vi "PD250 - PWM test.vi"(8 "Board Selector":T1, 10 "Message IN":string=" ", 11 "HMP4040 Channel Settings":T2={"CH1 Voltage"=24.0, "CH1 Current"=1.0, "CH1 Output"=TRUE, "CH2 Voltage"=24.0, "CH2 Current"=1.0, "CH2 Output"=TRUE, "CH3 Voltage"=24.0, "CH3 Current"=1.0, "CH3 Output"=TRUE, "CH4 Voltage"=24.0, "CH4 Current"=1.0, "CH4 Output"=TRUE, "Master Output"=TRUE} {"CH4 Current" format="%.3f"; "CH4 Voltage" format="%.3f"; "CH3 Current" format="%.3f"; "CH3 Voltage" format="%.3f"; "CH2 Current" format="%.3f"; "CH2 Voltage" format="%.3f"; "CH1 Current" format="%.3f"; "CH1 Voltage" format="%.3f"}) -> (0 "error out":errorcluster, 1 "Result (bool)":bool, 2 "Message OUT":string, 3 "ControlBoard OUT":refnum<visa-resource-name>)   [LabVIEW 2022 SP3]
uses:
  HMP4000 Communication/HMP4040_ChannelControl.ctl
  Serial Board Com/Board Select.ctl
  <vilib>/DAQmx/read.llb/DAQmx Read (Analog 1D Wfm NChan NSamp).vi
  <vilib>/DAQmx/miscellaneous.llb/DAQmx Fill In Error Info.vi
panel:
  in  "error in (no error) 2":errorcluster
  out "Analysis Leg":i32
  in  "Debug Mode":bool
  out "Waveforms":T3
  out "Active Leg":i32
  out "Result (color)":u32(colorbox)
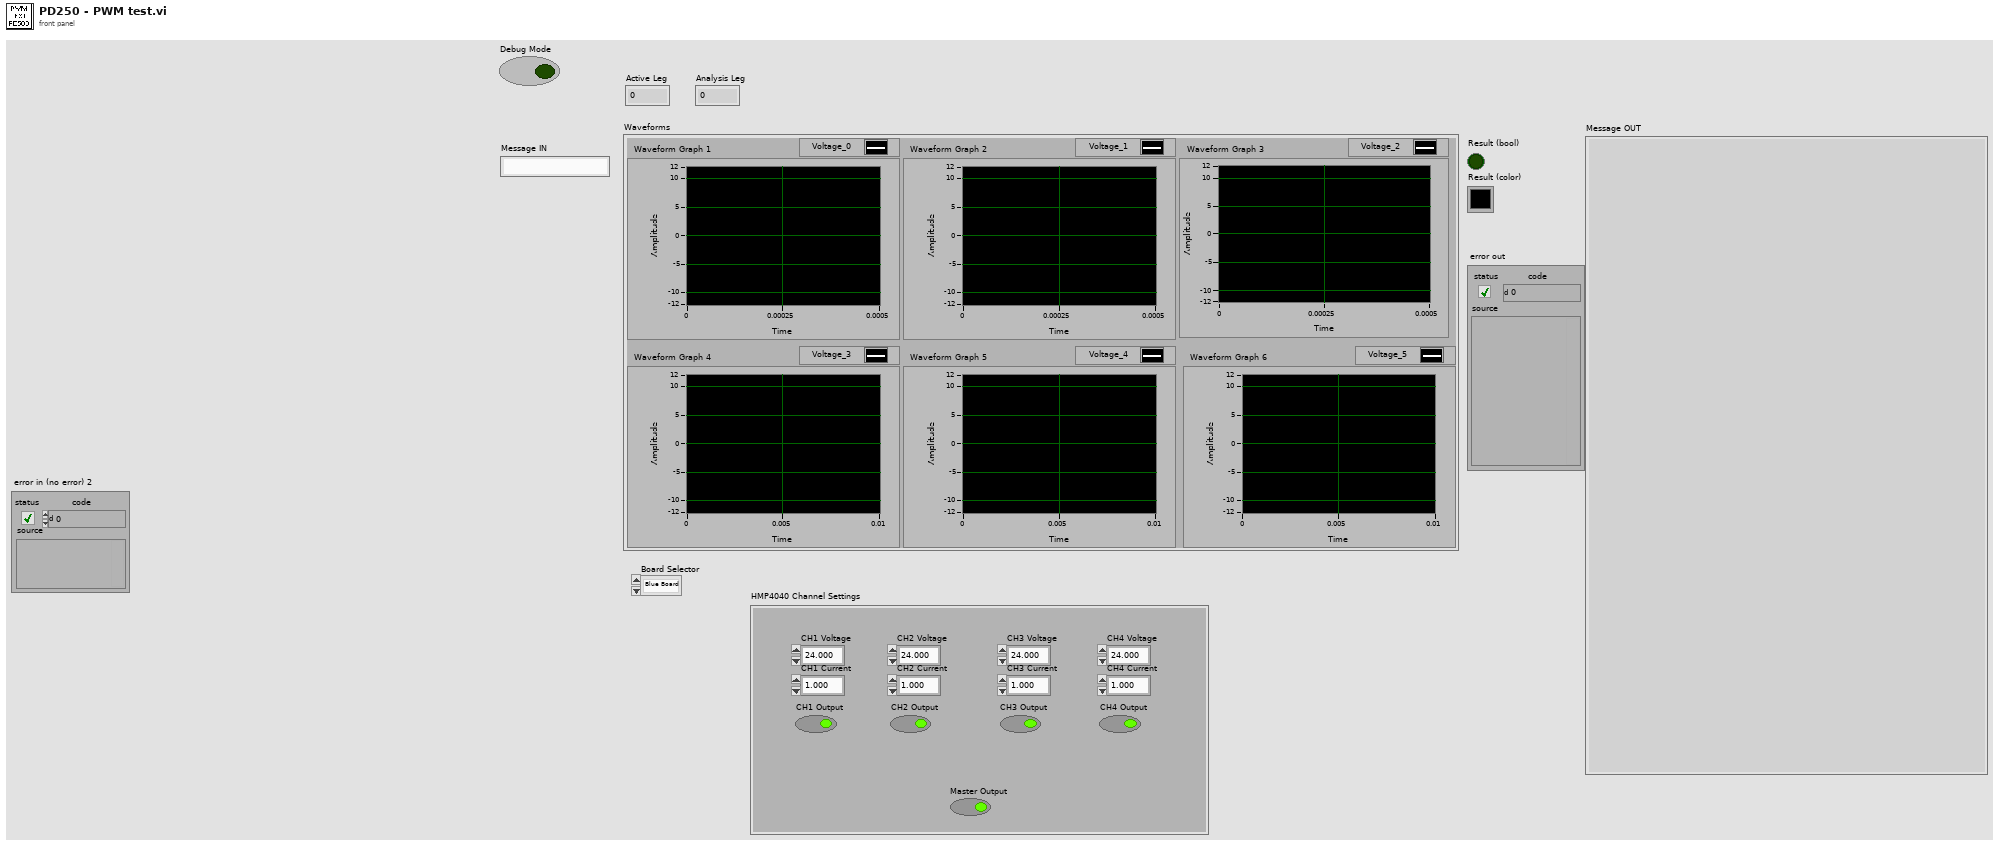
[diagram p1: front panel]
types:
  T1 = typedef "Board Select.ctl" = enum16{"Blue Board", "Green Board"}
  T2 = typedef "HMP4040_ChannelControl.ctl" = cluster{"CH1 Voltage":dbl, "CH1 Current":dbl, "CH1 Output":bool, "CH2 Voltage":dbl, "CH2 Current":dbl, "CH2 Output":bool, "CH3 Voltage":dbl, "CH3 Current":dbl, "CH3 Output":bool, "CH4 Voltage":dbl, "CH4 Current":dbl, "CH4 Output":bool, "Master Output":bool}
  T3 = cluster{"Waveform Graph 1":waveform(dbl), "Waveform Graph 2":waveform(dbl), "Waveform Graph 3":waveform(dbl), "Waveform Graph 4":waveform(dbl), "Waveform Graph 5":waveform(dbl), "Waveform Graph 6":waveform(dbl)}
  T4 = cluster{"data[0]":waveform(dbl), "data[1]":waveform(dbl), "data[2]":waveform(dbl), "data[3]":waveform(dbl), "data[4]":waveform(dbl), "data[5]":waveform(dbl)}
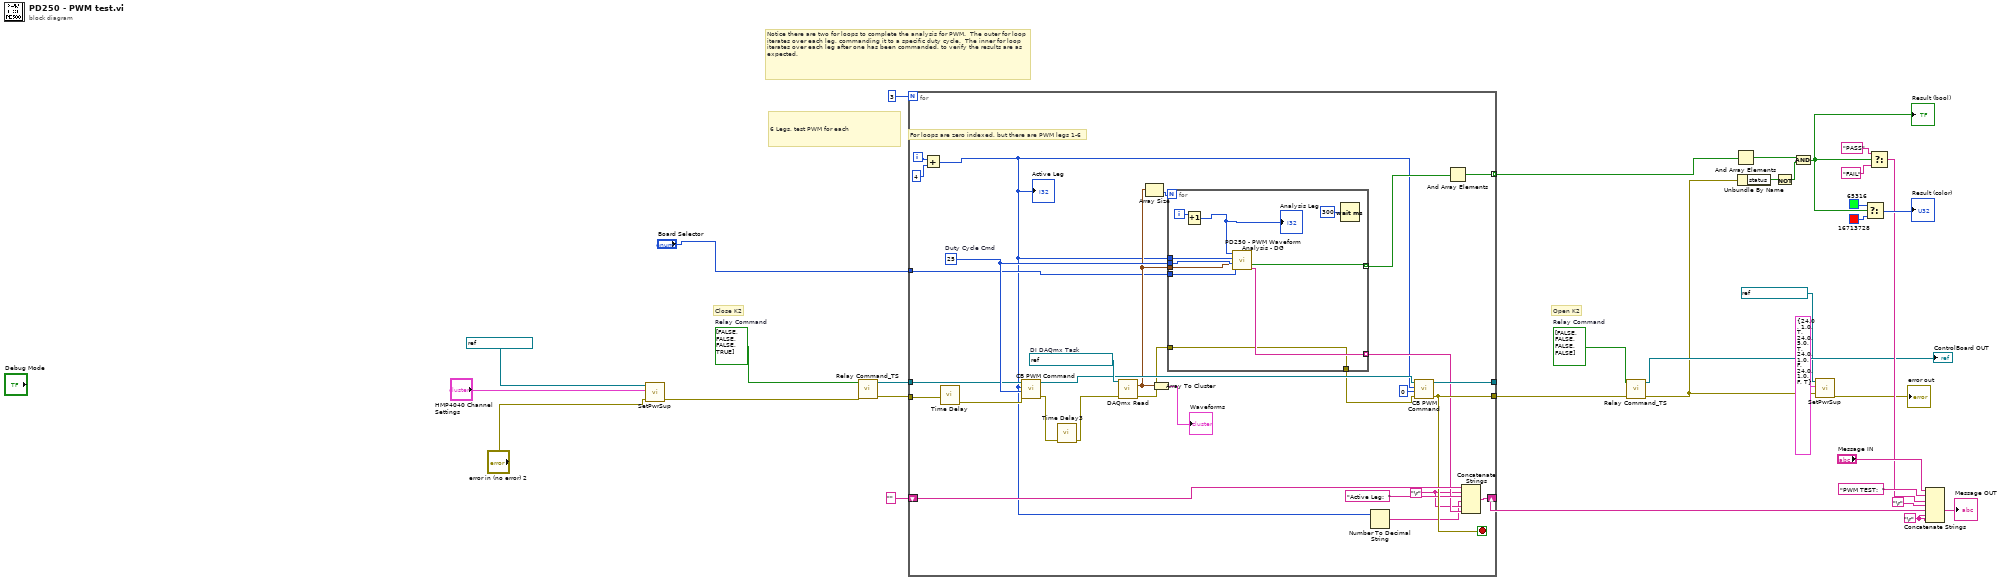
[diagram p0: block diagram]
diagram:
  w11 = bool[] [FALSE, FALSE, FALSE, TRUE]  # Relay Command
  w1 = bool[] [FALSE, FALSE, FALSE, FALSE]  # Relay Command
  w23 = "\r"
  # "Close K2"
  # "Open K2"
  # "Notice there are two for loops to complete the analysis for PWM.  The outer for loop iterates over each leg, commanding it to a specific duty cycle.  The inner for loop iterates over each leg after one has been commanded, to verify the results are as expected."
  # "6 Legs, test PWM for each"
  n1 = call "SetPwrSup.vi"("error in (no error)"="error in (no error) 2", "HMP4040 Channel Settings"="HMP4040 Channel Settings", "HMP4040 IN"=refnum<visa-resource-name> "HMP4040_FTS2" ("VISA resource name")) -> ("error out"=w7:errorcluster)  [unwired: 7 in, 1 out]
  n2 = call "Relay Command_TS.vi"("error in (no error)"=w7, "Relay Command"=w11) -> ("error out"=w12:errorcluster, "VISA Refnum out"=w13:refnum<visa-resource-name>)  [unwired: 8 in]
  n3 = for {
    N: 3 -> [_]
    tunnel: [w62] -> w34 mode=indexing
    shift-right: [w60] -> w21
    shift-left: "" -> [w59]
    tunnel: [w55] -> w15
    tunnel: [w50] -> _
    tunnel: w12 -> [w41]
    tunnel: w13 -> [w45]
    tunnel: "Board Selector" -> [w42]
    i -> [w36]
    stop <- w55 stop-if-true
    w47 = "\r"
    w56 = 25  # Duty Cycle Cmd
    w61 = refnum<k21> "FTS2_PWMInput_DG"  # DI DAQmx Task
    # "For loops are zero indexed, but there are PWM legs 1-6"
    n4 = Add(x=w36, y=4) -> (x+y=w37:i32)
    "Active Leg" <- w37
    n5 = call "Time Delay"("error in (no error)"=w41) -> ("error out"=w40:errorcluster)  [unwired: 10 in]
    n6 = call "CB PWM Command.vi"("error in (no error)"=w40, "Duty Cycle"=w56, "Leg"=w37, "VISA Refnum in"=w45) -> ("error out"=w44:errorcluster, "VISA Refnum out"=w57:refnum<visa-resource-name>)  [unwired: 5 in, 1 out]
    n7 = call "Time Delay3"("error in (no error)"=w44) -> ("error out"=w43:errorcluster)  [unwired: 10 in]
    n8 = call-poly <vilib>:"DAQmx Read.vi"("task/channels in"=w61, "error in"=w43) -> ("data"=w51:waveform(dbl)[], "error out"=w38:errorcluster)  [unwired: 11 in, 1 out]
    n9 = Array Size(array=w51) -> (size(s)=w52:i32)
    n10 = Array To Cluster(array=w51) -> (cluster=→"Waveforms":T4)
    n11 = for {
      N: w52 -> [_]
      tunnel: w56 -> [w72]
      tunnel: w51 -> [w71]
      tunnel: w37 -> [w70]
      tunnel: [w69] -> w53 mode=indexing
      tunnel: [w68] -> w48 mode=indexing
      tunnel: w42 -> [w67]
      tunnel: [w66] -> w39
      tunnel: w38 -> [w66]
      i -> [w64]
      n12 = Increment(x=w64) -> (x+1=w63:i32)
      "Analysis Leg" <- w63
      n13 = call "PD250 - PWM Waveform Analysis - DG.vi"("Analysis Leg"=w63, "Active Leg"=w70, "Duty Cycle"=w72, "Waveform"=w71, "Board Selector"=w67) -> ("Result (Boolean)"=w69:bool, "Message"=w68:string)  [unwired: 9 in]
      n14 = Wait (ms)(milliseconds to wait=u32 300) -> ()  [unwired: 1 out]
    }
    n15 = Number To Decimal String(number=w37) -> (decimal integer string=w46:string)  [unwired: 1 in]
    n16 = call "CB PWM Command.vi"("error in (no error)"=w39, "Duty Cycle"=0, "Leg"=w37, "VISA Refnum in"=w57) -> ("error out"=w55:errorcluster, "VISA Refnum out"=w50:refnum<visa-resource-name>)  [unwired: 5 in, 1 out]
    n17 = And Array Elements(Boolean array=w53) -> (logical AND=w62:bool)
    n18 = Concatenate Strings(w59, w47, "Active Leg:  ", w46, w47, w48) -> (w60:string)
  }
  n19 = call "Relay Command_TS.vi"("error in (no error)"=w15, "Relay Command"=w1) -> ("error out"=w4:errorcluster, "VISA Refnum out"=→"ControlBoard OUT":refnum<visa-resource-name>)  [unwired: 8 in]
  n20 = And Array Elements(Boolean array=w34) -> (logical AND=w24:bool)
  n21 = Unbundle By Name(w4) -> ("status"=w27:bool)
  n22 = Not(x=w27) -> (.not. x?=w26:bool)
  n23 = And(x=w24, y=w26) -> (x .and. y?=w25:bool)
  "Result (bool)" <- w25
  n24 = call "SetPwrSup.vi"("error in (no error)"=w4, "HMP4040 Channel Settings"=T2 {"CH1 Voltage"=24.0, "CH1 Current"=1.0, "CH1 Output"=TRUE, "CH2 Voltage"=24.0, "CH2 Current"=5.0, "CH2 Output"=TRUE, "CH3 Voltage"=24.0, "CH3 Current"=1.0, "CH3 Output"=FALSE, "CH4 Voltage"=24.0, "CH4 Current"=1.0, "CH4 Output"=FALSE, "Master Output"=TRUE}, "HMP4040 IN"=refnum<visa-resource-name> "HMP4040_FTS2" ("VISA resource name")) -> ("error out"=→"error out":errorcluster)  [unwired: 7 in, 1 out]
  n25 = Select(t=u32 65316 ("Result (color)"), s=w25, f=u32 16713728 ("Result (color)")) -> (s? t:f=→"Result (color)":u32)
  n26 = Select(t="PASS", s=w25, f="FAIL") -> (s? t:f=w16:string)
  n27 = Concatenate Strings("Message IN", "PWM TEST:  ", w16, "\r", w21, w23, w23) -> (→"Message OUT":string)
